vi "read_sensirion_from_arduino (sub-vi).vi"(8 "error in":errorcluster, 9 "expected num sensors (12)":i32=12, 10 "serial buffer in":string) -> (0 "error out":errorcluster, 2 "sensor data array":T1[](array[typedef]) {"temperature" scale=293.15..303.15 scale format="%#_3g"})   [LabVIEW 2021]
uses:
  controls/sensirion_flow_sensor_data.ctl
  type-defs/project_custom_error_codes_ring (type def).ctl
  <vilib>/regexp/Match Regular Expression.xnode
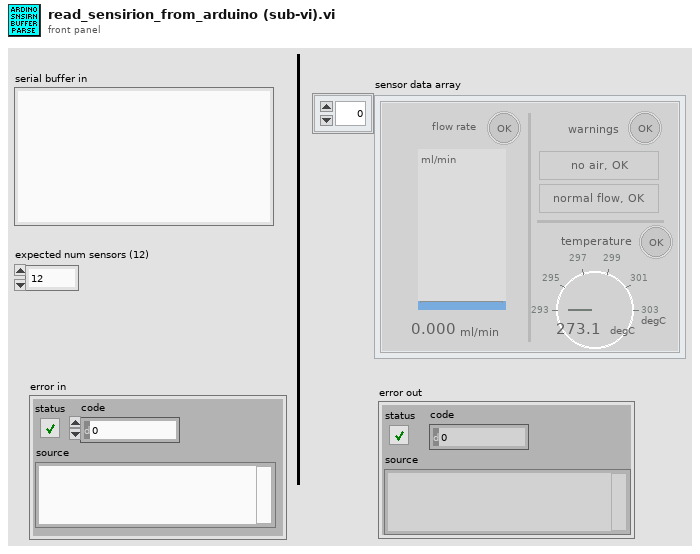
[diagram p1: front panel]
types:
  T1 = typedef "sensirion_flow_sensor_data.ctl" = cluster{"flow rate \n":dbl[unit], "flow val. status":bool, "temperature":dbl[unit], "temp. val status":bool, "air in line?":bool, "high flow?":bool, "flag. val status":bool}
  T2 = cluster{dbl[unit], "TRUE":bool, dbl[unit], "TRUE":bool, "FALSE":bool, "FALSE":bool, "TRUE":bool}[]
  T3 = typedef "project_custom_error_codes_ring (type def).ctl" = i32
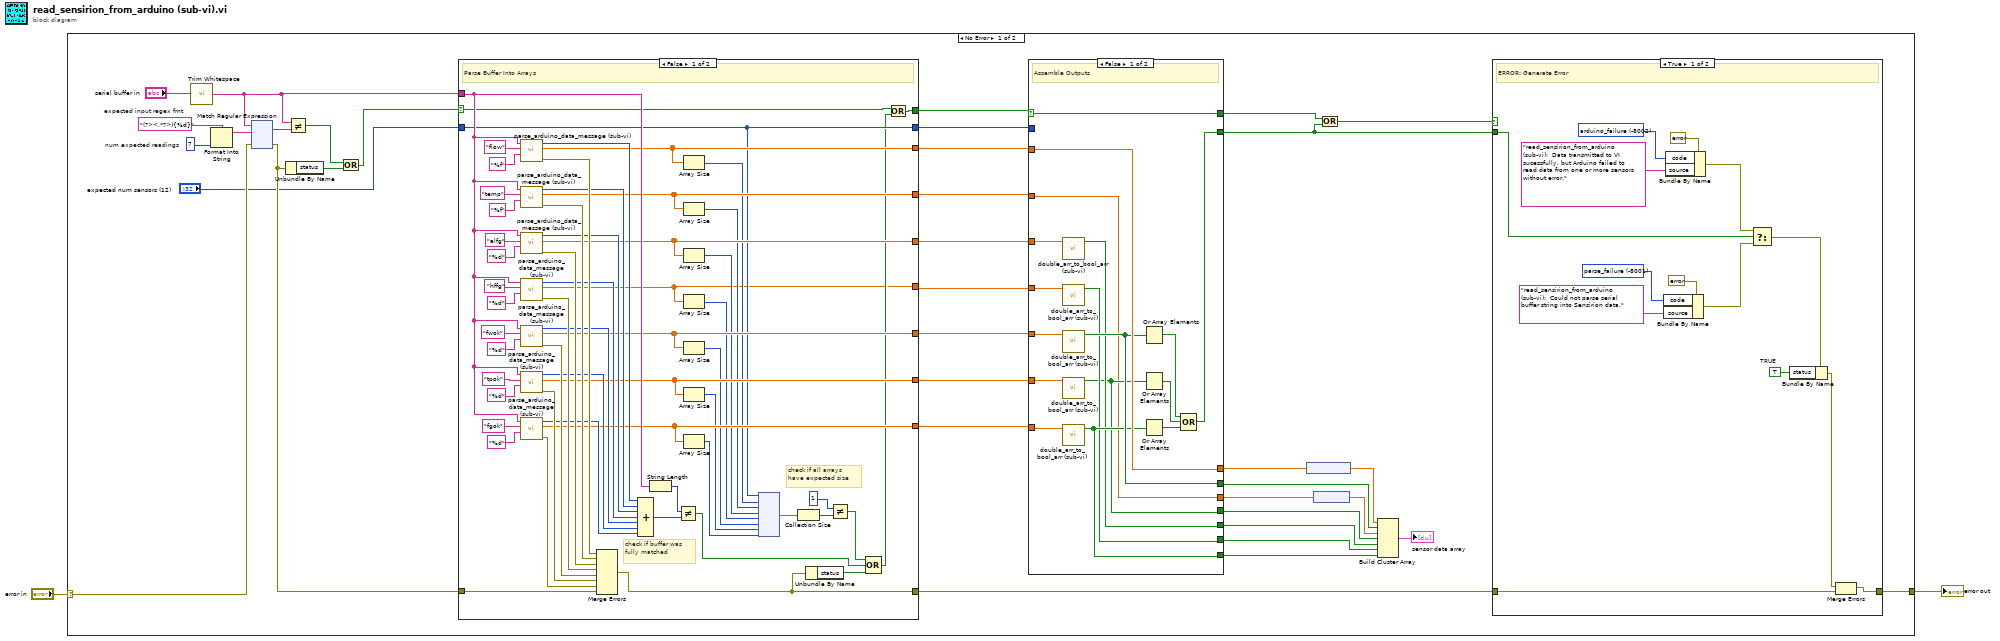
[diagram p0: block diagram]
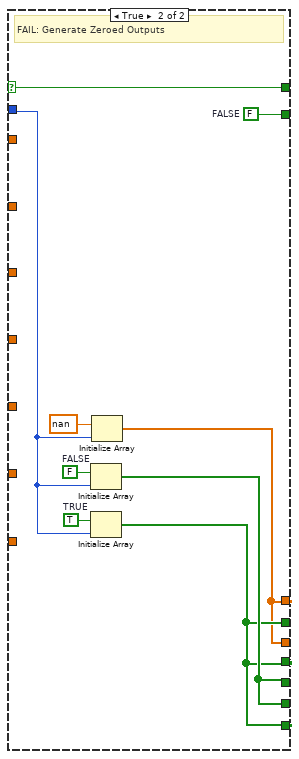
[diagram p3: hidden frame]
diagram:
  n1 = case shown="No Error" "error in" {
    selector: "error in" -> [w12 w257]
    tunnel: [w20 w257] -> w2
    frame No Error {
      w38 = 7  # num expected readings
      w37 = "(?><.*?>){%d}"  # expected input regex fmt
      n2 = call <vilib>:"Trim Whitespace.vi"("string"="serial buffer in") -> ("trimmed string"=w31:string)  [unwired: 1 in]
      n3 = Format Into String(format string=w37, w38) -> (resulting string=w36:string)  [unwired: 2 in, 1 out]
      n4 = xnode "Match Regular Expression"("input string"=w31, "regular expression"=w36, "error in"=w12) -> ("whole match"=w35:string, "error out"=w13:errorcluster)  [unwired: 3 in, 3 out]
      n5 = Unbundle By Name(w13) -> ("status"=w33:bool)
      n6 = Not Equal?(x=w31, y=w35) -> (x != y?=w34:bool)
      n7 = Or(x=w34, y=w33) -> (x .or. y?=w32:bool)
      n8 = case "Initial Buffer Processing" shown="False" w32 {
        selector: w32 -> [w89 w139]
        tunnel: w31 -> [w105 _]
        tunnel: w13 -> [w122 w137]
        tunnel: [w113 w137] -> w21
        tunnel: [w114 w139] -> w23
        tunnel: [w101 _] -> w27
        tunnel: [w102 _] -> w26
        tunnel: [w100 _] -> w28
        tunnel: [w80 _] -> w29
        tunnel: [w99 _] -> w30
        tunnel: [w98 _] -> w25
        tunnel: [w97 _] -> w24
        tunnel: "expected num sensors (12)" -> [w88 w138]
        tunnel: [w88 w138] -> w22
        frame False {
          # "check if buffer was \nfully matched"
          # "check if all arrays have expected size"
          # "Parse Buffer Into Arrays"
          n9 = call "parse_arduino_data_message (sub-vi).vi"("format string (%f)"="%f" ("input 1"), "data label"="flow" ("input 1"), "input string"=w105) -> ("error out"=w115:errorcluster, "array out"=w97:dbl[], "match length"=w112:i32)  [unwired: 6 in]
          n10 = call "parse_arduino_data_message (sub-vi).vi"("format string (%f)"="%f" ("input 1"), "data label"="temp" ("input 1"), "input string"=w105) -> ("error out"=w116:errorcluster, "array out"=w98:dbl[], "match length"=w111:i32)  [unwired: 6 in]
          n11 = call "parse_arduino_data_message (sub-vi).vi"("format string (%f)"="%d" ("input 1"), "data label"="alfg" ("input 1"), "input string"=w105) -> ("error out"=w117:errorcluster, "array out"=w99:dbl[], "match length"=w110:i32)  [unwired: 6 in]
          n12 = call "parse_arduino_data_message (sub-vi).vi"("format string (%f)"="%d" ("input 1"), "data label"="hffg" ("input 1"), "input string"=w105) -> ("error out"=w118:errorcluster, "array out"=w80:dbl[], "match length"=w109:i32)  [unwired: 6 in]
          n13 = call "parse_arduino_data_message (sub-vi).vi"("format string (%f)"="%d" ("input 1"), "data label"="fwok" ("input 1"), "input string"=w105) -> ("error out"=w119:errorcluster, "array out"=w100:dbl[], "match length"=w108:i32)  [unwired: 6 in]
          n14 = call "parse_arduino_data_message (sub-vi).vi"("format string (%f)"="%d" ("input 1"), "data label"="tpok" ("input 1"), "input string"=w105) -> ("error out"=w120:errorcluster, "array out"=w101:dbl[], "match length"=w107:i32)  [unwired: 6 in]
          n15 = call "parse_arduino_data_message (sub-vi).vi"("format string (%f)"="%d" ("input 1"), "data label"="fgok" ("input 1"), "input string"=w105) -> ("error out"=w121:errorcluster, "array out"=w102:dbl[], "match length"=w106:i32)  [unwired: 6 in]
          n16 = Merge Errors(w115, w116, w117, w118, w119, w120, w121, w122) -> (w113:errorcluster)
          n17 = Compound Arithmetic op=ADD(w112, w111, w110, w109, w108, w107, w106) -> (w104:i32)
          n18 = String Length(string=w105) -> (length=w103:i32)
          n19 = Not Equal?(x=w103, y=w104) -> (x != y?=w83:bool)
          n20 = Array Size(array=w97) -> (size(s)=w90:i32)
          n21 = Array Size(array=w98) -> (size(s)=w91:i32)
          n22 = Array Size(array=w99) -> (size(s)=w92:i32)
          n23 = Array Size(array=w80) -> (size(s)=w93:i32)
          n24 = Array Size(array=w100) -> (size(s)=w94:i32)
          n25 = Array Size(array=w101) -> (size(s)=w95:i32)
          n26 = Array Size(array=w102) -> (size(s)=w96:i32)
          n27 = node(w88, w90, w91, w92, w93, w94, w95, w96) -> (w87:set{i32})
          n28 = Collection Size(1:w87) -> (0:w86:i32)
          n29 = Unbundle By Name(w113) -> ("status"=w84:bool)
          n30 = Not Equal?(x=1, y=w86) -> (x != y?=w82:bool)
          n31 = Compound Arithmetic op=OR(w82, w83, w84) -> (w81:bool)
          n32 = Or(x=w89, y=w81) -> (x .or. y?=w114:bool)
        }
        frame True {
          # "FAIL: Pass on Default Arrays"
        }
      }
      n33 = case shown="False" w23 {
        selector: w23 -> [w65 w79]
        tunnel: w30 -> [w70 _]
        tunnel: w29 -> [w69 _]
        tunnel: w28 -> [w68 _]
        tunnel: w27 -> [w67 _]
        tunnel: w26 -> [w66 _]
        tunnel: w25 -> [w54 _]
        tunnel: w24 -> [w60 _]
        tunnel: w22 -> [_ w75]
        tunnel: [w65 w79] -> w8
        tunnel: [w61 w74] -> w7
        tunnel: [w60 w71] -> w6
        tunnel: [w59 w72] -> w19
        tunnel: [w54 w71] -> w18
        tunnel: [w55 w72] -> w17
        tunnel: [w56 w73] -> w16
        tunnel: [w57 w73] -> w15
        tunnel: [w58 w72] -> w14
        frame False {
          # "Assemble Outputs"
          n34 = call "double_arr_to_bool_arr (sub-vi).vi"("double array"=w70) -> ("bool array"=w56:bool[])  [unwired: 4 in]
          n35 = call "double_arr_to_bool_arr (sub-vi).vi"("double array"=w69) -> ("bool array"=w57:bool[])  [unwired: 4 in]
          n36 = call "double_arr_to_bool_arr (sub-vi).vi"("double array"=w68) -> ("bool array"=w59:bool[])  [unwired: 4 in]
          n37 = call "double_arr_to_bool_arr (sub-vi).vi"("double array"=w67) -> ("bool array"=w55:bool[])  [unwired: 4 in]
          n38 = call "double_arr_to_bool_arr (sub-vi).vi"("double array"=w66) -> ("bool array"=w58:bool[])  [unwired: 4 in]
          n39 = Or Array Elements(Boolean array=w59) -> (logical OR=w64:bool)
          n40 = Or Array Elements(Boolean array=w55) -> (logical OR=w63:bool)
          n41 = Or Array Elements(Boolean array=w58) -> (logical OR=w62:bool)
          n42 = Compound Arithmetic op=OR(w64, w63, w62) -> (w61:bool)
        }
        frame True {
          w74 = FALSE  # FALSE
          w76 = TRUE  # TRUE
          w77 = FALSE  # FALSE
          # "FAIL: Generate Zeroed Outputs"
          n43 = Initialize Array(w77, w75) -> (w73:bool[])
          n44 = Initialize Array(w76, w75) -> (w72:bool[])
          n45 = Initialize Array(nan, w75) -> (w71:dbl[])
        }
      }
      n46 = node(w6) -> (w5:dbl[unit][])
      n47 = node(w18) -> (w3:dbl[unit][])
      n48 = Or(x=w8, y=w7) -> (x .or. y?=w9:bool)
      n49 = Build Cluster Array(w5, w19, w3, w17, w16, w15, w14) -> (→"sensor data array":T2)
      n50 = case shown="True" w9 {
        tunnel: w21 -> [w52 w53]
        tunnel: [w51 w53] -> w20
        tunnel: w7 -> [w50 _]
        frame True {
          w40 = TRUE  # TRUE
          w44 = T3 -8001 items=["parse_failure"=-8001, "arduino_failure"=-8002] ("Ring")
          w49 = T3 -8002 items=["parse_failure"=-8001, "arduino_failure"=-8002] ("Ring")
          # "ERROR: Generate Error"
          n51 = Bundle By Name(cluster=errorcluster {"status"=FALSE, "code"=0, "source"=""} ("error constant"), "code"=w44, "source"="read_sensirion_from_arduino (sub-vi):  Could not parse serial buffer string into Sensirion data.") -> (w43:errorcluster)
          n52 = Bundle By Name(cluster=errorcluster {"status"=FALSE, "code"=0, "source"=""} ("error constant"), "code"=w49, "source"="read_sensirion_from_arduino (sub-vi):  Data transmitted to VI sucessfully, but Arduino failed to read data from one or more sensors without error.") -> (w42:errorcluster)
          n53 = Select(t=w42, s=w50, f=w43) -> (s? t:f=w41:errorcluster)
          n54 = Bundle By Name(cluster=w41, "status"=w40) -> (w39:errorcluster)
          n55 = Merge Errors(w39, w52) -> (w51:errorcluster)
        }
        frame False {
          # "No Error to Generate"
        }
      }
    }
    frame Error {
    }
  }
  "error out" <- w2
